vi "SolveMotor_Speed,Torque.vi"(8 "Reference Voltage (12)":dbl=12.0, 9 "Motor Characteristics":T2, 10 "Motor Torque":dbl, 11 "Motor Speed":dbl) -> (3 "Motor Data":T1)   [LabVIEW 2014]
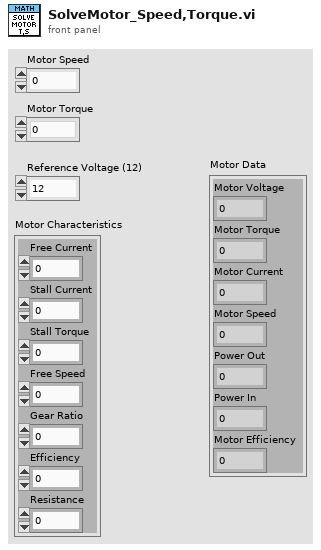
[diagram p1: front panel]
types:
  T1 = cluster{"Motor Voltage":dbl, "Motor Torque":dbl, "Motor Current":dbl, "Motor Speed":dbl, "Power Out":dbl, "Power In":dbl, "Motor Efficiency":dbl}
  T2 = cluster{"Free Current":dbl, "Stall Current":dbl, "Stall Torque":dbl, "Free Speed":dbl, "Gear Ratio":dbl, "Efficiency":dbl, "Resistance":dbl}
  T3 = cluster{"[0]":dbl, "[1]":dbl, "[2]":dbl, "[3]":dbl, "[4]":dbl, "[5]":dbl, "[6]":dbl}
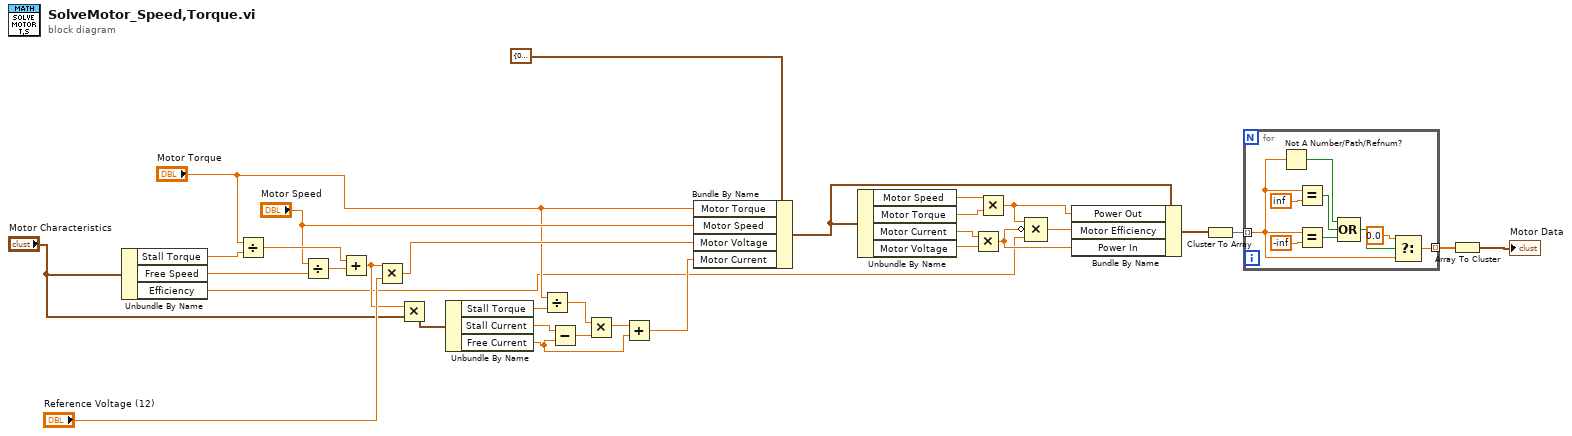
[diagram p0: block diagram]
diagram:
  n1 = Unbundle By Name("Motor Characteristics") -> ("Stall Torque"=w23:dbl, "Free Speed"=w22:dbl, "Efficiency"=w5:dbl)
  n2 = Divide(x="Motor Torque", y=w23) -> (x/y=w20:dbl)
  n3 = Divide(x="Motor Speed", y=w22) -> (x/y=w21:dbl)
  n4 = Add(x=w20, y=w21) -> (x+y=w16:dbl)
  n5 = Multiply(x=w16, y="Reference Voltage (12)") -> (x*y=w18:dbl)
  n6 = Multiply(x=w16, y="Motor Characteristics") -> (x*y=w14:T2)
  n7 = Unbundle By Name(w14) -> ("Stall Torque"=w13:dbl, "Stall Current"=w11:dbl, "Free Current"=w7:dbl)
  n8 = Divide(x="Motor Torque", y=w13) -> (x/y=w9:dbl)
  n9 = Subtract(x=w11, y=w7) -> (x-y=w10:dbl)
  n10 = Multiply(x=w9, y=w10) -> (x*y=w8:dbl)
  n11 = Add(x=w8, y=w7) -> (x+y=w6:dbl)
  n12 = Bundle By Name(cluster=T1 {"Motor Voltage"=0.0, "Motor Torque"=0.0, "Motor Current"=0.0, "Motor Speed"=0.0, "Power Out"=0.0, "Power In"=0.0, "Motor Efficiency"=0.0} ("Motor Data"), "Motor Torque"="Motor Torque", "Motor Speed"="Motor Speed", "Motor Voltage"=w18, "Motor Current"=w6) -> (w24:T1)
  n13 = Unbundle By Name(w24) -> ("Motor Speed"=w32:dbl, "Motor Torque"=w31:dbl, "Motor Current"=w29:dbl, "Motor Voltage"=w30:dbl)
  n14 = Multiply(x=w29, y=w30) -> (x*y=w26:dbl)
  n15 = Multiply(x=w32, y=w31) -> (x*y=w27:dbl)
  n16 = Compound Arithmetic op=MULTIPLY(w27, invert w26, w5) -> (w28:dbl)
  n17 = Bundle By Name(cluster=w24, "Power Out"=w27, "Motor Efficiency"=w28, "Power In"=w26) -> (w2:T1)
  n18 = Cluster To Array(cluster=w2) -> (array=w4:dbl[])
  n19 = for {
    tunnel: w4 -> [w38] mode=indexing
    tunnel: [w33] -> w3 mode=indexing
    n20 = Not A Number/Path/Refnum?(number/path/refnum=w38) -> (NaN/Path/Refnum?=w37:bool)
    n21 = Equal?(x=w38, y=inf) -> (x = y?=w35:bool)
    n22 = Equal?(x=w38, y=-inf) -> (x = y?=w36:bool)
    n23 = Compound Arithmetic op=OR(w37, w35, w36) -> (w34:bool)
    n24 = Select(t=0.0, s=w34, f=w38) -> (s? t:f=w33:dbl)
  }
  n25 = Array To Cluster(array=w3) -> (cluster=→"Motor Data":T3)
